vi "Send Configure Msg.vi"(8 "error in":errorcluster, 10 "digital generation":T1={"data channel list"="", "master clock channel list"="", "digital protocol settings"={"logic level"=enum."3.3 V", "PCM Data Configuration"={"Frame Sync Edge for Channel 0"=enum."Falling", "Channel Count Per Frame"=2, "Channel Length"=32, "Bit Depth"=24, "Channel 0 Offset"=1, "Endianness"=enum."MSB First", "Data Justification"=enum."Left Justified"}, "bit clock rate"=3025000.0, "master clock rate"=3025000.0, "clock mode"=enum."divided clock", "Frame Sync Clock Control"={"Frame Length"=64, "Frame Sync Pulse Width"=32, "Bit Clock Edge  Sync"=enum."Falling"}}, "signal parameters"={"cyclic signal"=[], "channel parameters"=[]}} {"digital protocol settings"."master clock rate" format="%.4p"; "digital protocol settings"."bit clock rate" format="%.4p"}, 11 "Qbus in":refnum<class "Qbus.lvclass">) -> (0 "error out":errorcluster, 3 "Qbus out":refnum<class "Qbus.lvclass">)   [LabVIEW 2021, in "DigitalAudioGenerationProcess.lvlib"]
uses:
  DigitalAudioGenerationProcess.lvlib
  <vilib>/addons/Qbus/Qbus.lvclass
  controls/digital generation settings.ctl
  controls/digital protocol settings.ctl
  <vilib>/PDM Acquisition Toolkit/host/Classes/Session/Controls/Logic Levels.ctl
  <vilib>/PDM Acquisition Toolkit/shared/controls/PCM Data Format Configuration.ctl
  <vilib>/PDM Acquisition Toolkit/shared/controls/Digital Edge.ctl
  <vilib>/PDM Acquisition Toolkit/shared/controls/PCM Bit Endianness.ctl
  <vilib>/PDM Acquisition Toolkit/shared/controls/PCM Data Justification.ctl
  <vilib>/PDM Acquisition Toolkit/shared/controls/clock mode.ctl
  <vilib>/PDM Acquisition Toolkit/shared/controls/PCM Frame Sync Control.ctl
  <vilib>/PDM Acquisition Toolkit/host/Classes/Tasks/I2S Output/Control/SignalProperties.ctl
  <vilib>/PDM Acquisition Toolkit/host/Classes/Channels/I2S Ouput/Controls/GenerationChannelProperties.ctl
  <vilib>/PDM Acquisition Toolkit/host/Classes/Session/DecoderSession.lvclass
  <vilib>/PDM Acquisition Toolkit/shared/PDM Shared.lvlib
  controls/AudioGenTypeDefs.lvlib
  <vilib>/PDM Acquisition Toolkit/host/Classes/Channels/I2S Ouput/I2S Output Channel.lvclass
  <vilib>/PDM Acquisition Toolkit/host/Classes/Tasks/I2S Output/I2S Output Task.lvclass
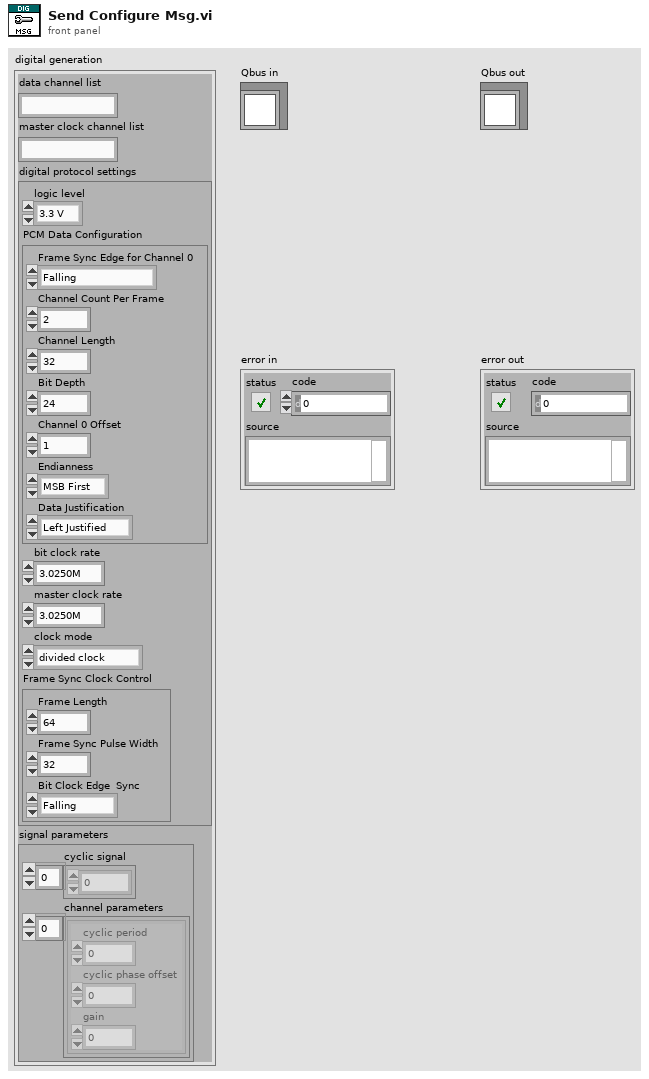
[diagram p1: front panel]
types:
  T1 = typedef "AudioGenTypeDefs.lvlib/digital generation settings.ctl" = cluster{"data channel list":string, "master clock channel list":string, "digital protocol settings":T2, "signal parameters":T10}
  T2 = typedef "AudioGenTypeDefs.lvlib/digital protocol settings.ctl" = cluster{"logic level":T3, "PCM Data Configuration":T4, "bit clock rate":sgl, "master clock rate":sgl, "clock mode":T8, "Frame Sync Clock Control":T9}
  T3 = typedef "PDM Acquisition Class Library.lvlib/DecoderSession.lvclass/Logic Levels.ctl" = enum16{"3.3 V", "1.8 V", "1.2 V"}
  T4 = typedef "PDM Shared.lvlib/PCM Data Format Configuration.ctl" = cluster{"Frame Sync Edge for Channel 0":T5, "Channel Count Per Frame":u8, "Channel Length":u16, "Bit Depth":u8, "Channel 0 Offset":u16, "Endianness":T6, "Data Justification":T7}
  T5 = typedef "PDM Shared.lvlib/Digital Edge.ctl" = enum8{"Rising", "Falling"}
  T6 = typedef "PDM Shared.lvlib/PCM Bit Endianness.ctl" = enum16{"MSB First", "LSB First"}
  T7 = typedef "PDM Shared.lvlib/PCM Data Justification.ctl" = enum16{"Left Justified", "Right Justified"}
  T8 = typedef "PDM Shared.lvlib/clock mode.ctl" = enum16{"divided clock", "DDS"}
  T9 = typedef "PDM Shared.lvlib/PCM Frame Sync Control.ctl" = cluster{"Frame Length":u16, "Frame Sync Pulse Width":u16, "Bit Clock Edge  Sync":T5}
  T10 = typedef "PDM Acquisition Class Library.lvlib/I2S Output Task.lvclass/SignalProperties.ctl" = cluster{"cyclic signal":dbl[], "channel parameters":T11[]}
  T11 = typedef "PDM Acquisition Class Library.lvlib/I2S Output Channel.lvclass/GenerationChannelProperties.ctl" = cluster{"cyclic period":dbl, "cyclic phase offset":dbl, "gain":dbl}
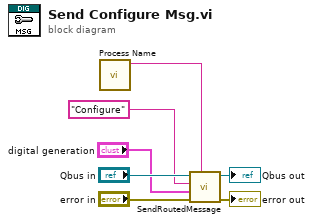
[diagram p0: block diagram]
diagram:
  n1 = call "Process Name.vi"() -> ("process name"=w2:string)  [unwired: 11 in]
  n2 = call <vilib>:"SendRoutedMessage.vi"("listener process"=w2, "error in (no error)"="error in", "message value"="digital generation", "message name"="Configure", "Qbus in"="Qbus in") -> ("error in (no error)"=→"error out":errorcluster, "Qbus out"=→"Qbus out":refnum<class "Qbus.lvclass">)  [unwired: 5 in]
